vi "Set Key Value (U32).vi"(5 "Key name":string, 6 "Key value":u32, 7 "Section name":string, 8 "error in (no error)":errorcluster, 9 "Create key? [T]":bool=TRUE, 10 "Create section? [T]":bool=TRUE, 11 "Carya Config in":refnum<class "Carya Config.lvclass">) -> (0 "error out":errorcluster, 1 "Created key?":bool, 2 "Created session?":bool, 3 "Carya Config out":refnum<class "Carya Config.lvclass">, 4 "Value written?":bool)   [LabVIEW 2013, in "Carya Config.lvclass"]
doc: "Copyright 2018, Carya Automatisering, Wiebe Walstra."
uses:
  Carya Config.lvclass
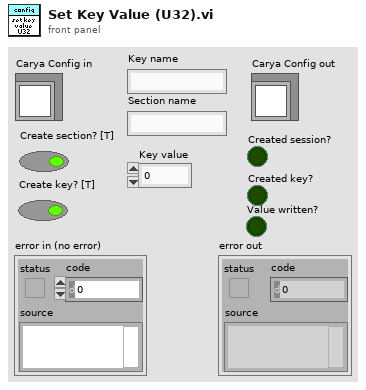
[diagram p1: front panel]
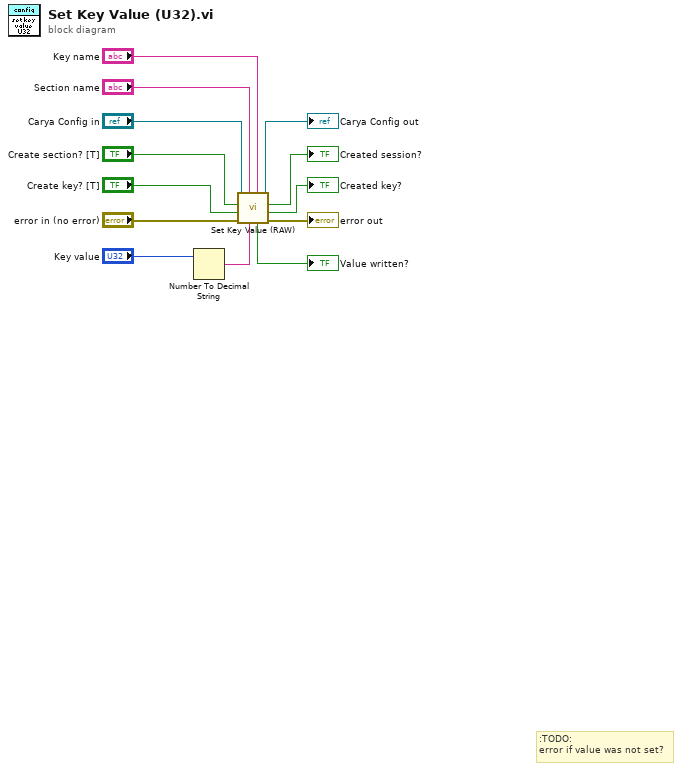
[diagram p0: block diagram]
diagram:
  # ":TODO:\nerror if value was not set?"
  n1 = Number To Decimal String(number="Key value") -> (decimal integer string=w2:string)  [unwired: 1 in]
  n2 = call-dynamic "Set Key Value (RAW).vi"("Key name"="Key name", "Key value"=w2, "Section name"="Section name", "error in (no error)"="error in (no error)", "Create key? [T]"="Create key? [T]", "Create section? [T]"="Create section? [T]", "Carya Config in"="Carya Config in") -> ("error out"=→"error out":errorcluster, "Created key?"=→"Created key?":bool, "Created session?"=→"Created session?":bool, "Carya Config out"=→"Carya Config out":refnum<class "Carya Config.lvclass">, "Value written?"=→"Value written?":bool)
